vi "set speed.vi"(10 "Speed":u8(slide) scale=0.0..250.0, 11 "Array":T1[](array[typedef]) {"Data" format="%.0x"}) -> (3 "Array 2":T1[](array[typedef]) {"Data" format="%.0x"})   [LabVIEW 2021, in "uCanDriver.lvlib" / "uCAN.lvclass"]
uses:
  uCAN.lvclass
  typedefs/frame.ctl
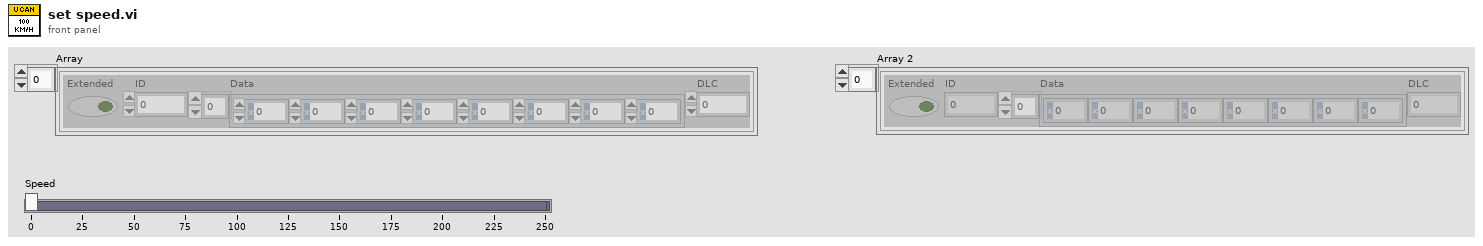
[diagram p1: front panel]
types:
  T1 = typedef "uCanDriver.lvlib/uCAN.lvclass/frame.ctl" = cluster{"Extended":bool, "ID":u32, "Data":u8[], "DLC":u8}
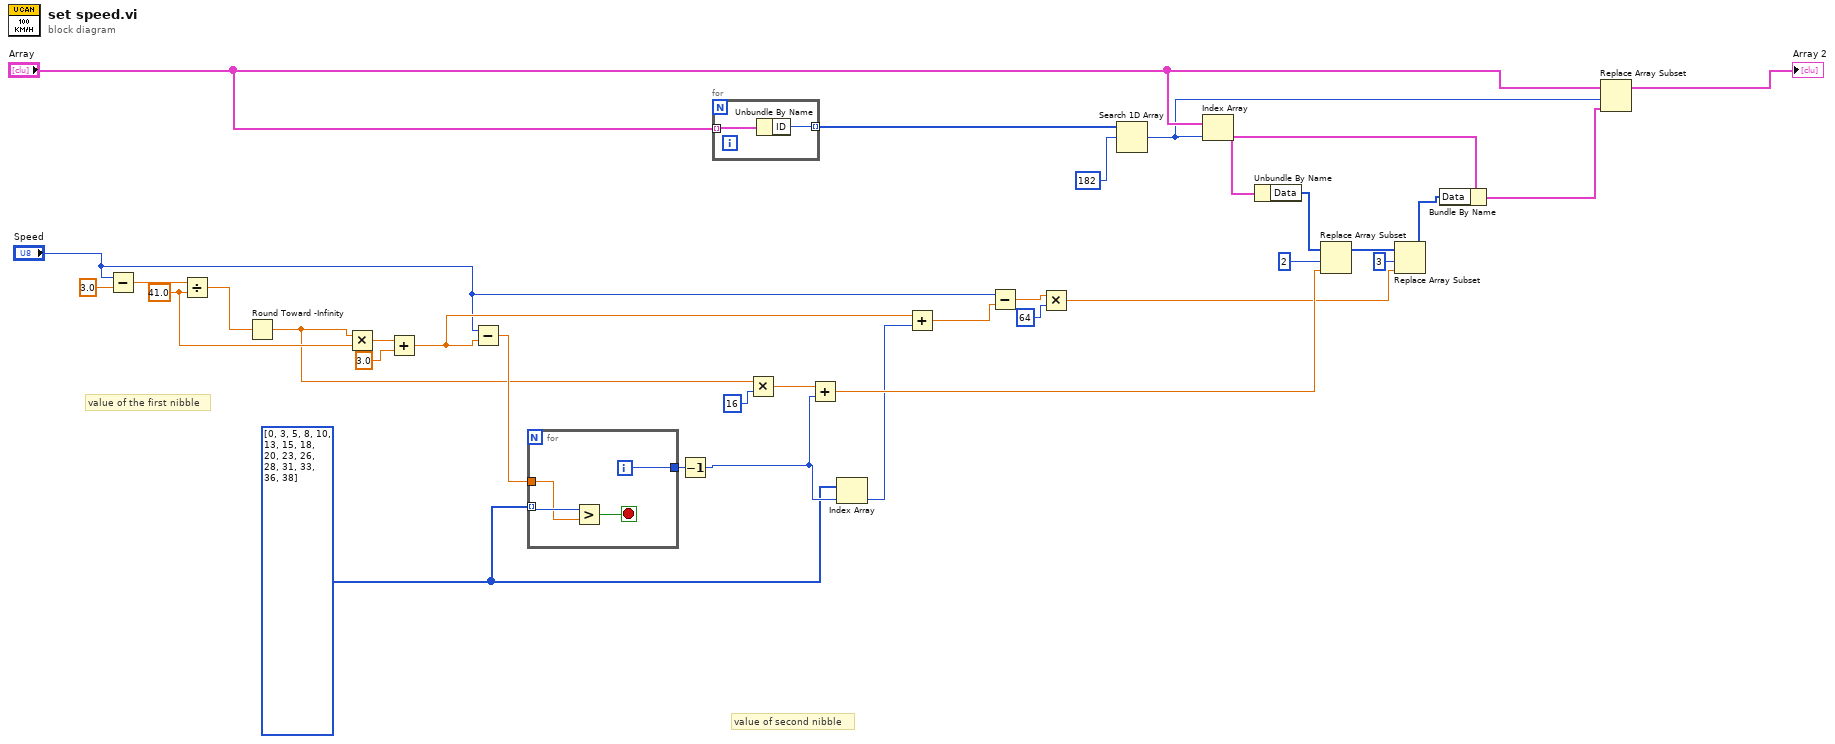
[diagram p0: block diagram]
diagram:
  w1 = i32[] [0, 3, 5, 8, 10, 13, 15, 18, 20, 23, 26, 28, 31, 33, 36, 38]
  w18 = 41.0 ("y")
  # "value of second nibble"
  # "value of the first nibble"
  n1 = Subtract(x="Speed", y=3.0) -> (x-y=w20:dbl)
  n2 = Divide(x=w20, y=w18) -> (x/y=w19:dbl)
  n3 = Round Toward -Infinity(1:w19) -> (0:w13:dbl)
  n4 = Multiply(x=w13, y=w18) -> (x*y=w17:dbl)
  n5 = Add(x=w17, y=3.0) -> (x+y=w9:dbl)
  n6 = Subtract(x="Speed", y=w9) -> (x-y=w15:dbl)
  n7 = for {
    tunnel: w1 -> [w37] mode=indexing
    tunnel: w15 -> [w36]
    tunnel: [w34] -> w14
    i -> [w34]
    stop <- w35 stop-if-true
    n8 = Greater?(x=w37, y=w36) -> (0:w35:bool)
  }
  n9 = Decrement(x=w14) -> (x-1=w3:i32)
  n10 = for {
    tunnel: "Array" -> [w39] mode=indexing
    tunnel: [w38] -> w31 mode=indexing
    n11 = Unbundle By Name(w39) -> ("ID"=w38:u32)
  }
  n12 = Multiply(x=w13, y=u8 16 ("unsigned 8bit integer")) -> (x*y=w11:dbl)
  n13 = Add(x=w11, y=w3) -> (x+y=w10:dbl)
  n14 = Index Array(array=w1, index=w3) -> (element=w2:i32)
  n15 = Add(x=w9, y=w2) -> (x+y=w8:dbl)
  n16 = Subtract(x="Speed", y=w8) -> (x-y=w5:dbl)
  n17 = Multiply(x=w5, y=u8 64 ("unsigned 8bit integer")) -> (x*y=w4:dbl)
  n18 = Search 1D Array(1D array=w31, element=u32 182) -> (index of element=w29:i32)  [unwired: 1 in]
  n19 = Index Array(array="Array", index=w29) -> (element=w33:T1)
  n20 = Unbundle By Name(w33) -> ("Data"=w25:u8[])
  n21 = Replace Array Subset(array=w25, new element=w10, index=2) -> (w24:u8[])
  n22 = Replace Array Subset(array=w24, new element=w4, index=3) -> (w23:u8[])
  n23 = Bundle By Name(cluster=w33, "Data"=w23) -> (w27:T1)
  n24 = Replace Array Subset(array="Array", new element=w27, index=w29) -> (→"Array 2":T1[])
